vi "CleanUp.vi"(11 "Python Code":string="import hub\nimport utime\n\nspeed = 0\ndata = []\nX = hub.port.A.motor\nsonic_sensor = hub.port.B.device\nsonic_sensor.mode(0)\nsonic_sensor.get()[0]\n​\nfor speed in range(40,91,5):\n    X.run_to_position(90,50)\n    utime.sleep(.5)\n    dist = 10000\n    X.run_to_position(-90,speed)\n    for i in range(100):\n        utime.sleep(0.01)\n        d = sonic_sensor.get()[0]\n        dist = dist if dist < d else d\n    X.run_to_position(90,50)\n    print(speed,dist/2.54)\n    data.append((speed,dist/2.54))\n    utime.sleep(3)\n\nabcdefghijklmnopqrstuvwxyz1234567890-=][';/.,~!@#$%^&*()_+|}{POIUYTREWQASDFGHJKL:\"?><MNBVCXZ`") -> (3 "spreadsheet string":string="import hub\nimport utime\n\nspeed = 0\ndata = []\nX = hub.port.A.motor\nsonic_sensor = hub.port.B.device\nsonic_sensor.mode(0)\nsonic_sensor.get()[0]\n\nfor speed in range(40,91,5):\n    X.run_to_position(90,50)\n    utime.sleep(.5)\n    dist = 10000\n    X.run_to_position(-90,speed)\n    for i in range(100):\n        utime.sleep(0.01)\n        d = sonic_sensor.get()[0]\n        dist = dist if dist < d else d\n    X.run_to_position(90,50)\n    print(speed,dist/2.54)\n    data.append((speed,dist/2.54))\n    utime.sleep(3)\n\nabcdefghijklmnopqrstuvwxyz1234567890-=][';/.,~!@#$%^&*()_+|}{POIUYTREWQASDFGHJKL:\"?><MNBVCXZ`\n")   [LabVIEW 2022 SP3]
uses:
  <vilib>/Utility/error.llb/Trim Whitespace One-Sided.vi
panel:
  out "string":string="​"
  out "characters removed":u8[](array[numeric])=[226, 128, 139]
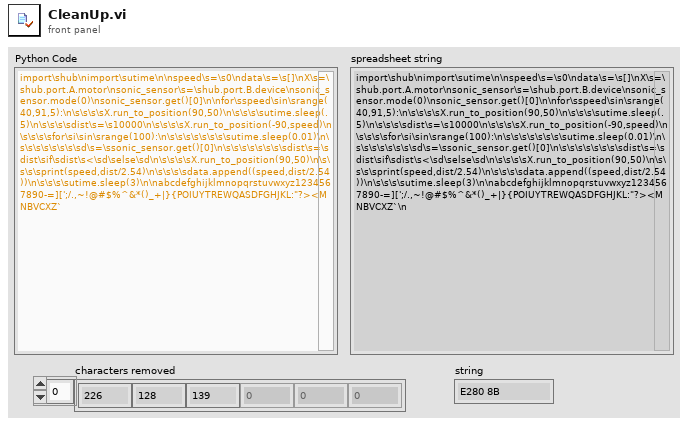
[diagram p1: front panel]
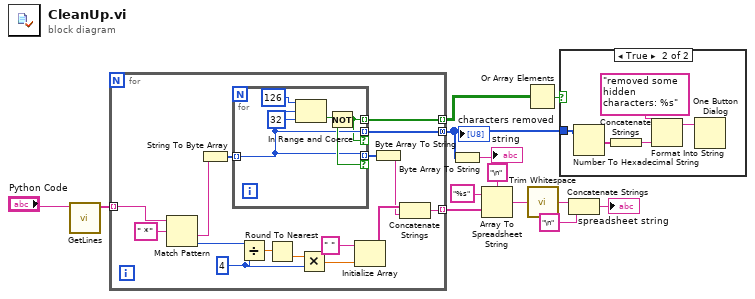
[diagram p0: block diagram]
diagram:
  n1 = call "GetLines.vi"("String"="Python Code") -> ("Array"=w5:string[])  [unwired: 10 in]
  n2 = for {
    tunnel: w5 -> [w29] mode=indexing
    tunnel: [w20] -> w10 mode=indexing
    tunnel: [w15] -> w4 mode=indexing
    tunnel: [w14] -> w1 mode=concatenating
    w24 = 4 ("y")
    n3 = Match Pattern(string=w29, regular expression=" *") -> (after substring=w19:string, offset past match=w27:i32)  [unwired: 1 in, 2 out]
    n4 = String To Byte Array(string=w19) -> (unsigned byte array=w18:u8[])
    n5 = for {
      tunnel: [w31] -> w17 mode=indexing if=w32
      tunnel: w18 -> [w31] mode=indexing
      tunnel: [w30] -> w15 mode=indexing
      tunnel: [w31] -> w14 mode=indexing if=w30
      n6 = In Range and Coerce(upper limit=u8 126, x=w31, lower limit=u8 32) -> (In Range?=w32:bool)  [unwired: 1 out]
      n7 = Not(x=w32) -> (.not. x?=w30:bool)
    }
    n8 = Divide(x=w27, y=w24) -> (x/y=w26:dbl)
    n9 = Round To Nearest(number=w26) -> (nearest integer value=w25:dbl)
    n10 = Multiply(x=w25, y=w24) -> (x*y=w23:dbl)
    n11 = Initialize Array(" " ("delimiter (Tab)"), w23) -> (w21:string[])
    n12 = Byte Array To String(unsigned byte array=w17) -> (string=w16:string)
    n13 = Concatenate Strings(w21, w16) -> (w20:string)
  }
  "characters removed" <- w1
  n14 = Byte Array To String(unsigned byte array=w1) -> (string=→"string":string)
  n15 = Array To Spreadsheet String(delimiter (Tab)="\n", array=w10, 3:"%s" ("format string")) -> (spreadsheet string=w13:string)
  n16 = Or Array Elements(Boolean array=w4) -> (logical OR=w3:bool)
  n17 = call <vilib>:"Trim Whitespace.vi"("string"=w13) -> ("trimmed string"=w9:string)  [unwired: 1 in]
  n18 = case shown="True" w3 {
    tunnel: w1 -> [_ w39]
    frame False {
    }
    frame True {
      n19 = Number To Hexadecimal String(2:w39) -> (0:w36:string[])  [unwired: 1 in]
      n20 = Concatenate Strings(w36) -> (w35:string)
      n21 = Format Into String(format string="removed some hidden characters: %s" ("message"), w35) -> (resulting string=w37:string)  [unwired: 2 in, 1 out]
      n22 = One Button Dialog(message=w37) -> ()  [unwired: 1 in, 1 out]
    }
  }
  n23 = Concatenate Strings(w9, "\n" ("delimiter (Tab)")) -> (→"spreadsheet string":string)
